vi "test_DB.vi"() -> ()   [LabVIEW 2015]
uses:
  BERTTA.dll
panel:
  out "save data":dbl
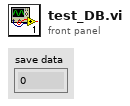
[diagram p1: front panel]
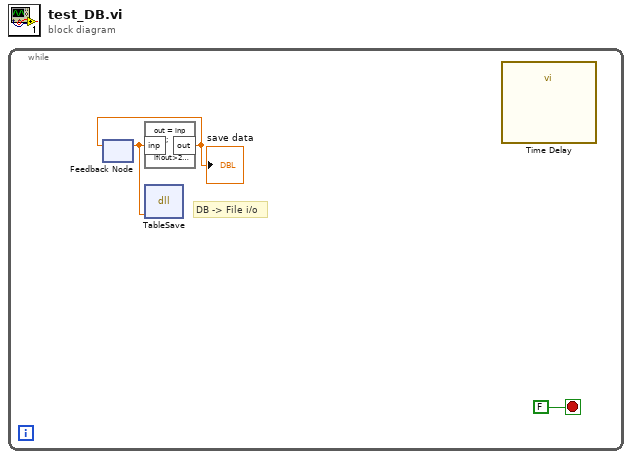
[diagram p0: block diagram]
diagram:
  n1 = while {
    stop <- FALSE stop-if-true
    # "DB -> File i/o"
    n2 = feedback #1() -> (w1:dbl)  [unwired: 1 in]
    n3 = formula code="out = inp + 1;\n\nif(out>20) out = 0;"("inp"=w1) -> ("out"=w2:dbl)
    "save data" <- w2
    n4 = feedback-in #1(w2) -> ()
    n5 = dll-call lib="C:/Users/xlaraser/Documents/Visual Studio 2017/Projects/Bertta/BERTTA/Debug/BERTTA.dll" fn="TableSave"("exec"=w1) -> ()  [unwired: 5 in, 2 out]
    n6 = call "Time Delay"() -> ()  [unwired: 11 in, 1 out]
  }
